vi "Add Value without TS.vi"(8 "Error In":errorcluster, 10 "Value":dbl, 11 "BNT_XtGraph in":refnum<class "BNT_XtGraph.lvclass">) -> (0 "Error Out":errorcluster, 3 "BNT_XtGraph out":refnum<class "BNT_XtGraph.lvclass">)   [LabVIEW 2018, in "BNT_XtGraph.lvlib" / "BNT_XtGraph.lvclass"]
doc: "Add actual value with time <b>now</b> to history."
uses:
  BNT_XtGraph.lvclass
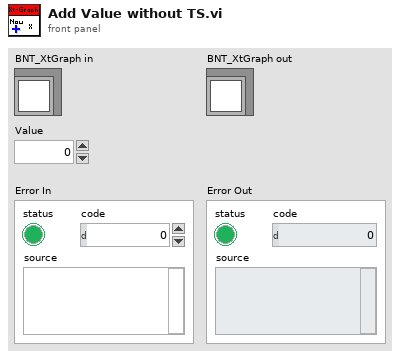
[diagram p1: front panel]
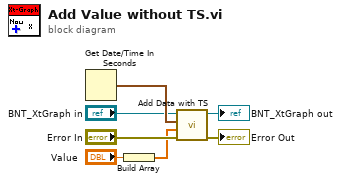
[diagram p0: block diagram]
diagram:
  n1 = Get Date/Time In Seconds() -> (seconds since 1Jan1904=w7:timestamp)
  n2 = Build Array("Value") -> (w1:dbl[])
  n3 = call "Add Data with TS.vi"("Error In"="Error In", "Values"=w1, "Time Stamp"=w7, "BNT_XtGraph in"="BNT_XtGraph in") -> ("Error Out"=→"Error Out":errorcluster, "BNT_XtGraph out"=→"BNT_XtGraph out":refnum<class "BNT_XtGraph.lvclass">)  [unwired: 6 in]
